vi "CountNumbers.vi"(10 "Array in":dbl[][](array[numeric]), 11 "Array 3":u8[](array[numeric])) -> (3 "Array out":dbl[][](array[numeric]))   [LabVIEW 2015]
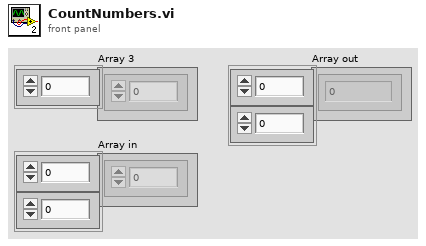
[diagram p1: front panel]
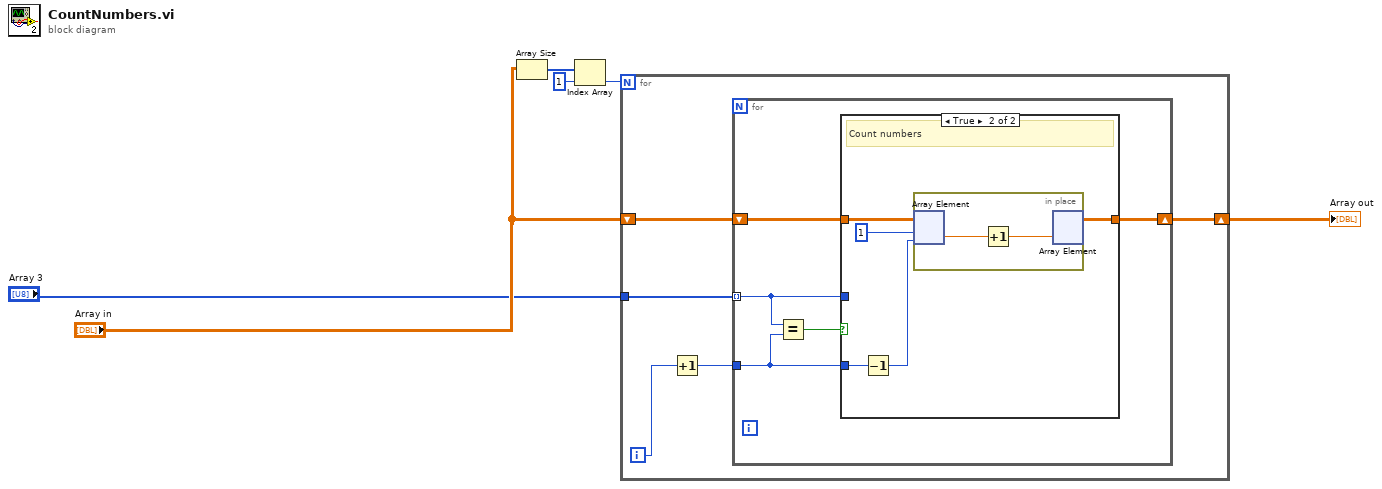
[diagram p0: block diagram]
diagram:
  n1 = Array Size(array="Array in") -> (size(s)=w2:i32[])
  n2 = Index Array(array=w2, index=1) -> (element=w4:i32)
  n3 = for {
    N: w4 -> [_]
    tunnel: "Array 3" -> [w8]
    shift-right: [w7] -> w6
    shift-left: "Array in" -> [w9]
    i -> [w11]
    n4 = Increment(x=w11) -> (x+1=w10:i32)
    n5 = for {
      tunnel: w10 -> [w15]
      tunnel: w8 -> [w12] mode=indexing
      shift-right: [w13] -> w7
      shift-left: w9 -> [w14]
      n6 = Equal?(x=w12, y=w15) -> (x = y?=w16:bool)
      n7 = case shown="True" w16 {
        tunnel: w15 -> [_ w21]
        tunnel: w12 -> [_ _]
        tunnel: w14 -> [w17 w22]
        tunnel: [w17 w20] -> w13
        frame False {
        }
        frame True {
          # "Count numbers"
          n8 = Decrement(x=w21) -> (x-1=w18:i32)
          n9 = in-place {
            n10 = in-place-array #1(w22, 1, w18) -> (w24:dbl)
            n11 = Increment(x=w24) -> (x+1=w23:dbl)
            n12 = in-place-array #1(w23) -> (w20:dbl[][])  [unwired: 2 out]
          }
        }
      }
    }
  }
  "Array out" <- w6
